vi "PEAK_Can_Write.vi"(5 "CAN Handle":T1, 7 "MSG type":enum8{"STD", "RTR", "XTD", "XTD RTR", "STATUS"}(ring), 8 "errin":errorcluster, 9 "CAN Data":u8[](array[numeric]) format="%x", 10 "DLC (8)":u8=8, 11 "Identifier":u32=1921 format="%x") -> (0 "errout":errorcluster)   [LabVIEW 2020, in "PEAK_lib_ALEX.lvlib"]
uses:
  <userlib>/Alex_Peak_lib/PEAK_lib_ALEX.lvlib
  <vilib>/nican/nican.llb/xobjhandle.ctl
  <userlib>/PCAN Basic/Controls/CAN MSG Cluster.ctl
  Users/Admin_Process/Desktop/Nouveau dossier (2)/C/Program Files (x86)/National Instruments/LabVIEW 2020/user.lib/PCAN Basic/PCANBasic.lvlib
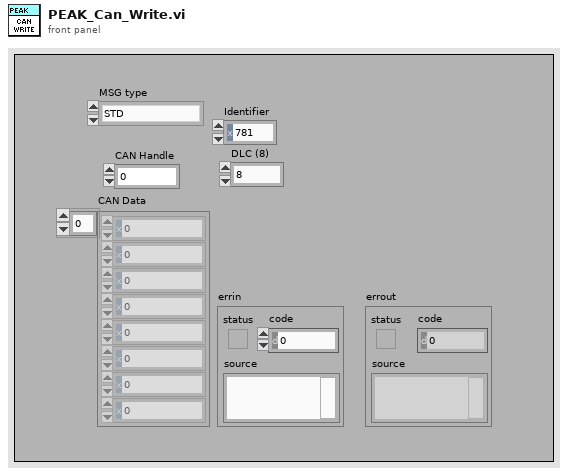
[diagram p1: front panel]
types:
  T1 = typedef "xobjhandle.ctl" = u32
  T2 = typedef "PCANBasic.lvlib/CAN MSG Cluster.ctl" = cluster{"ID":u32, "MSG type":enum8{"STD", "RTR", "XTD", "XTD RTR", "STATUS"}, "LEN":i8, "DATA":u8[]}
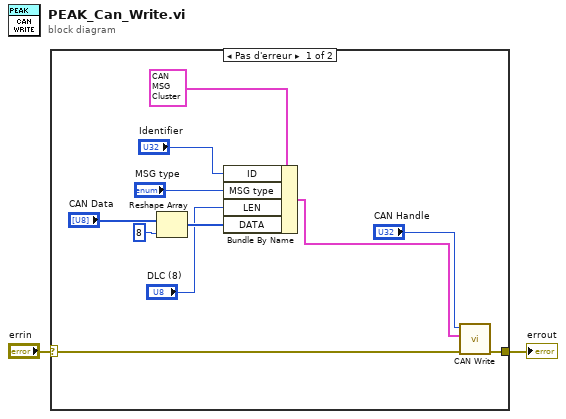
[diagram p0: block diagram]
diagram:
  n1 = case shown="Pas d'erreur" "errin" {
    selector: "errin" -> [w3 w14]
    tunnel: [w9 w14] -> w1
    frame No Error {
      n2 = Reshape Array("CAN Data", 8 ("taille de la dimension")) -> (w7:u8[])
      n3 = Bundle By Name(cluster=T2 {"ID"=0, "MSG type"=enum."STD", "LEN"=0, "DATA"=[0, 0, 0, 0, 0, 0, 0, 0]} ("CAN_Message"), "ID"="Identifier", "MSG type"="MSG type", "LEN"="DLC (8)", "DATA"=w7) -> (w11:T2)
      n4 = call <userlib>:"CAN Write.vi"("error in (no error)"=w3, "CAN_Message"=w11, "Channel"="CAN Handle") -> ("error out"=w9:errorcluster)  [unwired: 7 in, 1 out]
    }
    frame Error {
    }
  }
  "errout" <- w1
